vi "LabVIEW Measurement UI - Get Parameter.vi"(8 "error in":errorcluster, 11 "Measurement Client Wrapper in":refnum<class "Measurement Client Wrapper.lvclass">) -> (0 "error out":errorcluster, 1 "UI Indicator Details[]":T1[](array[typedef]), 2 "UI Control Details[]":T1[](array[typedef]), 3 "Measurement Client Wrapper":refnum<class "Measurement Client Wrapper.lvclass">)   [LabVIEW 2020, in "Measurement Client Wrapper.lvclass"]
uses:
  Measurement Client Wrapper.lvclass
  Typedefs/Control UI MetaData.ctl
  <vilib>/Utility/Data Type/Type Definitions/Data Type.ctl
  Typedefs/Measurement DataType.ctl
  Measurement Client Wrapper.lvclass/Measurement Client Wrapper.ctl
  <vilib>/Utility/Data Type/NI_Data Type.lvlib
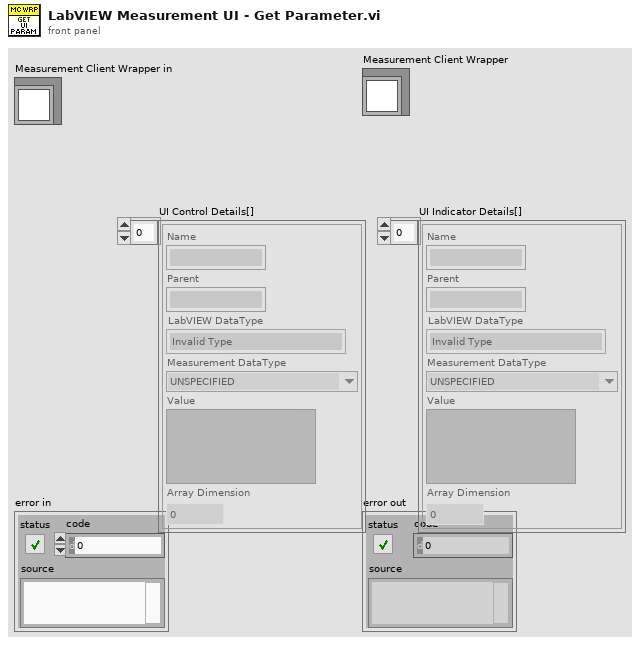
[diagram p1: front panel]
types:
  T1 = typedef "Measurement Client Wrapper.lvclass/Control UI MetaData.ctl" = cluster{"Name":string, "Parent":string, "LabVIEW DataType":T2, "Measurement DataType":T3, "Value":variant, "Array Dimension":i32}
  T2 = typedef "NI_Data Type.lvlib/Data Type.ctl" = enum8{"Invalid Type", "Void", "I8", "I16", "I32", "I64", "U8", "U16", "U32", "U64", "Single Float", "Double Float", "Extended Float", "Single Complex", "Double Complex", "Extended Complex", "Enum U8", "Enum U16", "Enum U32", "Enum U64", "Single Float With Unit", "Double Float With Unit", "Extended Float With Unit", "Single Complex with Unit", "Double Complex with Unit", "Extended Complex with Unit", "Boolean", "String", "Path", "Picture", "Tag", "Array", "Cluster", "Variant", "LV Variant", "Waveform", "Timestamp", "Digital Waveform", "Digital Data", "ExpressData", "Refnum", "External Data", "VI", "Poly VI", "LabVIEW Class Instance", "Fixed Point", "Set Collection", "Map Collection"}
  T3 = typedef "Measurement Client Wrapper.lvclass/Measurement DataType.ctl" = enum16{"UNSPECIFIED", "BOOL", "DOUBLE", "FLOAT", "INT32", "INT64", "STRING", "UINT32", "UINT64"}
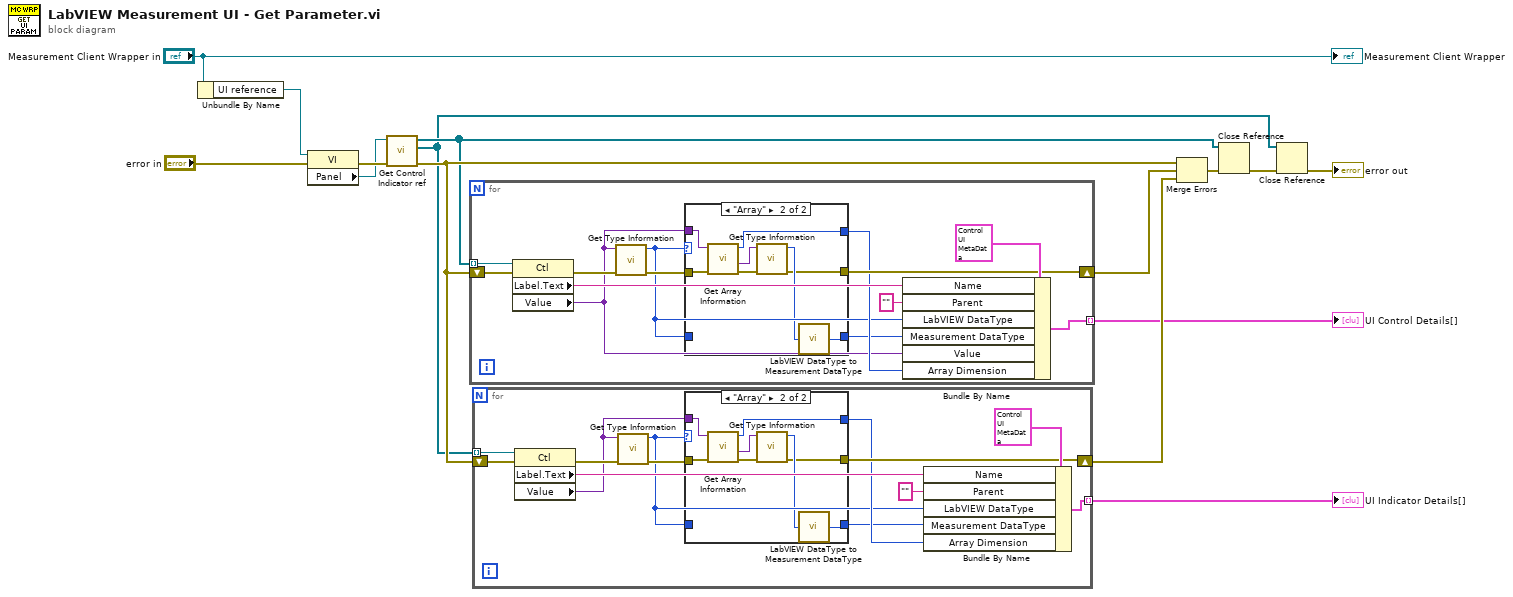
[diagram p0: block diagram]
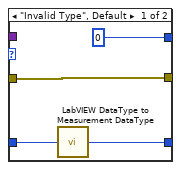
[diagram p2: hidden frame]
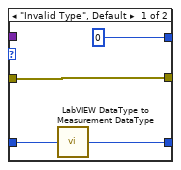
[diagram p3: hidden frame]
diagram:
  n1 = Unbundle By Name("Measurement Client Wrapper in") -> ("UI reference"=w1:refnum<vi>)
  n2 = property class="VI"(reference=w1, error in="error in") -> (error out=w14:errorcluster, "Panel"=w13:refnum<vi>)  [unwired: 1 out]
  n3 = call "Get Control Indicator ref.vi"("error in"=w14, "panel refnum"=w13) -> ("error out"=w12:errorcluster, "Indicators[]"=w6:refnum<vi>[], "Controls[]"=w8:refnum<vi>[])  [unwired: 7 in]
  n4 = for {
    tunnel: w8 -> [w28] mode=indexing
    shift-right: [w20] -> w9
    shift-left: w12 -> [w27]
    tunnel: [w22] -> w4 mode=indexing
    n5 = property class="Ctl"(reference=w28, error in=w27) -> (error out=w26:errorcluster, "Label.Text"=w24:string, "Value"=w18:variant)  [unwired: 1 out]
    n6 = call <vilib>:"Get Type Information.vi"("error in (no error)"=w26, "variant"=w18) -> ("error out"=w21:errorcluster, "type"=w17:T2)  [unwired: 5 in, 3 out]
    n7 = case shown="\"Array\"" w17 {
      tunnel: w21 -> [w32 w40]
      tunnel: [w32 w33] -> w20
      tunnel: [0 ("number of dimensions") w39] -> w19
      tunnel: w18 -> [_ w38]
      tunnel: w17 -> [w30 _]
      tunnel: [w29 w35] -> w16
      frame "Invalid Type", Default {
        n8 = call "LabVIEW DataType to Measurement DataType.vi"("LabVIEW type"=w30) -> ("Measurement DataType"=w29:T3)
      }
      frame "Array" {
        n9 = call <vilib>:"Get Array Information.vi"("error in (no error)"=w40, "variant"=w38) -> ("error out"=w34:errorcluster, "array element data type"=w37:variant, "number of dimensions"=w39:i32)  [unwired: 6 in, 1 out]
        n10 = call <vilib>:"Get Type Information.vi"("error in (no error)"=w34, "variant"=w37) -> ("error out"=w33:errorcluster, "type"=w36:T2)  [unwired: 5 in, 3 out]
        n11 = call "LabVIEW DataType to Measurement DataType.vi"("LabVIEW type"=w36) -> ("Measurement DataType"=w35:T3)
      }
    }
    n12 = Bundle By Name(cluster=T1 {"Name"="", "Parent"="", "LabVIEW DataType"=enum."Invalid Type", "Measurement DataType"=enum."UNSPECIFIED", "Value"=variant, "Array Dimension"=0} ("Control Details"), "Name"=w24, "Parent"="", "LabVIEW DataType"=w17, "Measurement DataType"=w16, "Value"=w18, "Array Dimension"=w19) -> (w22:T1)
  }
  "UI Control Details[]" <- w4
  n13 = for {
    tunnel: w6 -> [w53] mode=indexing
    shift-right: [w45] -> w10
    shift-left: w12 -> [w52]
    tunnel: [w47] -> w3 mode=indexing
    n14 = property class="Ctl"(reference=w53, error in=w52) -> (error out=w48:errorcluster, "Label.Text"=w50:string, "Value"=w42:variant)  [unwired: 1 out]
    n15 = call <vilib>:"Get Type Information.vi"("error in (no error)"=w48, "variant"=w42) -> ("error out"=w46:errorcluster, "type"=w41:T2)  [unwired: 5 in, 3 out]
    n16 = case shown="\"Array\"" w41 {
      tunnel: w46 -> [w57 w65]
      tunnel: [w57 w58] -> w45
      tunnel: [0 ("number of dimensions") w64] -> w44
      tunnel: w42 -> [_ w63]
      tunnel: w41 -> [w55 _]
      tunnel: [w54 w60] -> w43
      frame "Invalid Type", Default {
        n17 = call "LabVIEW DataType to Measurement DataType.vi"("LabVIEW type"=w55) -> ("Measurement DataType"=w54:T3)
      }
      frame "Array" {
        n18 = call <vilib>:"Get Array Information.vi"("error in (no error)"=w65, "variant"=w63) -> ("error out"=w59:errorcluster, "array element data type"=w62:variant, "number of dimensions"=w64:i32)  [unwired: 6 in, 1 out]
        n19 = call <vilib>:"Get Type Information.vi"("error in (no error)"=w59, "variant"=w62) -> ("error out"=w58:errorcluster, "type"=w61:T2)  [unwired: 5 in, 3 out]
        n20 = call "LabVIEW DataType to Measurement DataType.vi"("LabVIEW type"=w61) -> ("Measurement DataType"=w60:T3)
      }
    }
    n21 = Bundle By Name(cluster=T1 {"Name"="", "Parent"="", "LabVIEW DataType"=enum."Invalid Type", "Measurement DataType"=enum."UNSPECIFIED", "Value"=variant, "Array Dimension"=0} ("Control Details"), "Name"=w50, "Parent"="", "LabVIEW DataType"=w41, "Measurement DataType"=w43, "Array Dimension"=w44) -> (w47:T1)
  }
  "UI Indicator Details[]" <- w3
  n22 = Merge Errors(w12, w9, w10) -> (w11:errorcluster)
  n23 = Close Reference(reference=w8, error in (no error)=w11) -> (error out=w7:errorcluster)
  n24 = Close Reference(reference=w6, error in (no error)=w7) -> (error out=→"error out":errorcluster)
  "Measurement Client Wrapper" <- "Measurement Client Wrapper in"
